vi "Artificial Horizon.vi"(7 "Fixed Camera Position":bool=TRUE, 8 "error in \n(no error)":errorcluster, 9 "Heading":dbl(slide) scale=-360.0..360.0, 10 "Roll":dbl(slide) scale=-180.0..180.0, 11 "Pitch":dbl(slide) scale=-90.0..90.0) -> (0 "error out":errorcluster, 3 "reference out":refnum<vi>(3d-picture))   [LabVIEW 2011]
doc: "Artificial Horizon.VI\n\nRecieves Pitch Roll and Head, and using a 3D picture control Builds up an artifical horizon similar to that found in aircraft for example."
uses:
  <vilib>/Utility/miscctls.llb/LV3DPointTypeDef.ctl
  <vilib>/picture/3D Picture Control/NI_3D Picture Control.lvlib
panel:
  in  "Stop Button":bool
  # "Disabled"
  # "Enabled"
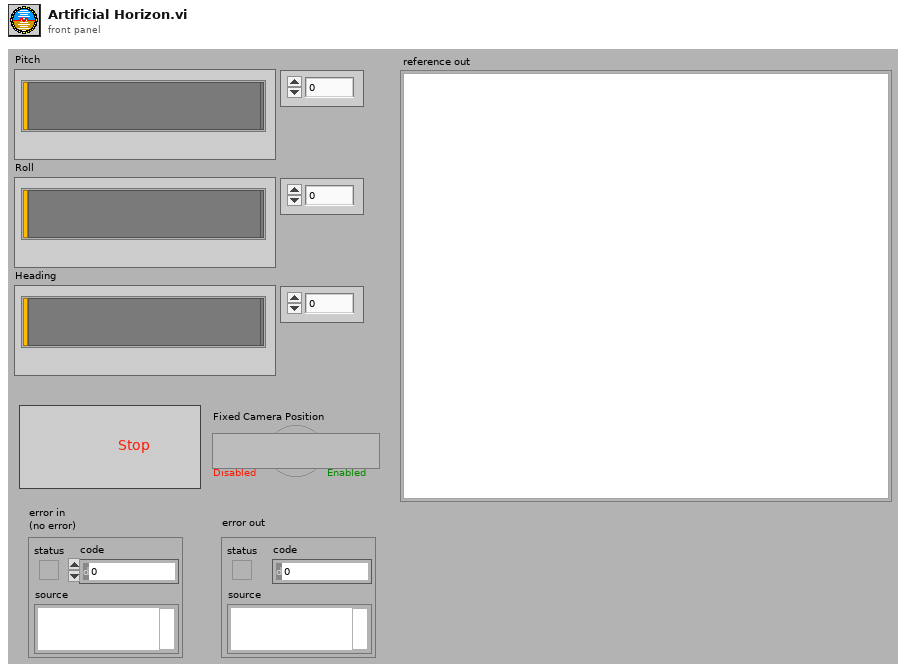
[diagram p1: front panel]
types:
  T1 = enum16{"None", "Spherical", "Flying", "Oriented"}
  T2 = typedef "LV3DPointTypeDef.ctl" = cluster{"X":sgl, "Y":sgl, "Z":sgl}
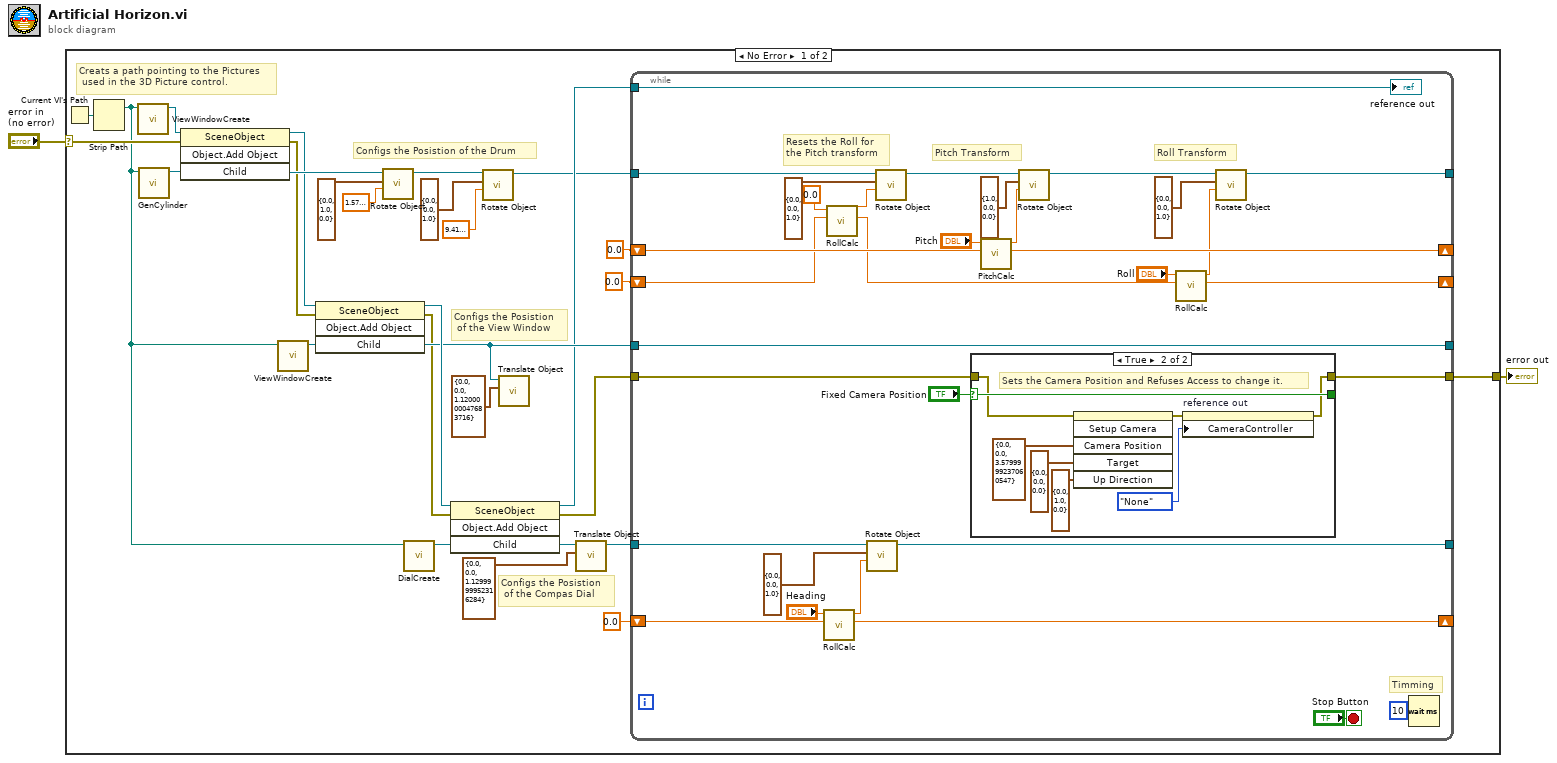
[diagram p0: block diagram]
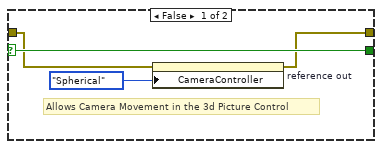
[diagram p2: hidden frame]
diagram:
  n1 = case shown="No Error" "error in \n(no error)" {
    selector: "error in \n(no error)" -> [w11 w76]
    tunnel: [w10 w76] -> w1
    frame No Error {
      # "Configs the Posistion\n of the Compas Dial"
      # "Configs the Posistion\n of the View Window"
      # "Configs the Posistion of the Drum"
      # "Creats a path pointing to the Pictures\n used in the 3D Picture control."
      n2 = Current VI's Path() -> (path=w6:path)
      n3 = Strip Path(path=w6) -> (stripped path=w4:path)  [unwired: 1 out]
      n4 = call "ViewWindowCreate.vi"("Solid Horizon Path.PNG"=w4) -> ("SceneObject out"=w5:refnum<vi>)  [unwired: 10 in]
      n5 = call "GenCylinder.vi"("Solid Horizon Path.PNG"=w4) -> ("SceneObject out"=w29:refnum<vi>)  [unwired: 10 in]
      n6 = invoke class="SceneObject" method="Object.Add Object"(reference=w5, error in=w11, "Child"=w29) -> (reference out=w15:refnum<vi>, error out=w9:errorcluster, "Child"=w22:refnum<vi>)  [unwired: 1 in, 1 out]
      n7 = call "ViewWindowCreate.vi"("Solid Horizon Path.PNG"=w4) -> ("SceneObject out"=w3:refnum<vi>)  [unwired: 10 in]
      n8 = invoke class="SceneObject" method="Object.Add Object"(reference=w15, error in=w9, "Child"=w3) -> (reference out=w31:refnum<vi>, error out=w8:errorcluster, "Child"=w25:refnum<vi>)  [unwired: 1 in, 1 out]
      n9 = call <vilib>:"Rotate Object.vi"("Angle"=sgl 1.5799999 ("Angle 2"), "Axis"=cluster{"X":sgl, "Y":sgl, "Z":sgl} {"X"=0.0, "Y"=1.0, "Z"=0.0} ("Axis 2"), "Scene.Object In"=w22) -> ("Scene.Object Out"=w21:refnum<vi>)  [unwired: 7 in, 1 out]
      n10 = call "DialCreate.vi"("Solid Horizon Path.PNG"=w4) -> ("SceneObject out"=w30:refnum<vi>)  [unwired: 10 in]
      n11 = invoke class="SceneObject" method="Object.Add Object"(reference=w31, error in=w8, "Child"=w30) -> (reference out=w16:refnum<vi>, error out=w7:errorcluster, "Child"=w26:refnum<vi>)  [unwired: 1 in, 1 out]
      n12 = call <vilib>:"Rotate Object.vi"("Angle"=sgl 9.419999 ("Angle 3"), "Axis"=cluster{"X":sgl, "Y":sgl, "Z":sgl} {"X"=0.0, "Y"=0.0, "Z"=1.0} ("Axis 3"), "Scene.Object In"=w21) -> ("Scene.Object Out"=w12:refnum<vi>)  [unwired: 7 in, 1 out]
      n13 = call <vilib>:"Translate Object.vi"("Translation"=cluster{"X":sgl, "Y":sgl, "Z":sgl} {"X"=0.0, "Y"=0.0, "Z"=1.12} ("Translation 4"), "Scene.Object In"=w25) -> ()  [unwired: 8 in, 2 out]
      n14 = call <vilib>:"Translate Object.vi"("Translation"=cluster{"X":sgl, "Y":sgl, "Z":sgl} {"X"=0.0, "Y"=0.0, "Z"=1.13} ("Translation 5"), "Scene.Object In"=w26) -> ("Scene.Object Out"=w14:refnum<vi>)  [unwired: 8 in, 1 out]
      n15 = while {
        tunnel: w25 -> [w58]
        tunnel: w16 -> [w62]
        tunnel: w12 -> [w61]
        shift-right: [w54] -> _
        shift-left: 0.0 ("y") -> [w55]
        shift-right: [w56] -> _
        shift-left: 0.0 ("y") -> [w52]
        tunnel: [w58] -> _
        tunnel: [w57] -> _
        tunnel: w14 -> [w50]
        shift-right: [w49] -> _
        shift-left: 0.0 ("y") -> [w51]
        tunnel: [w48] -> _
        tunnel: w7 -> [w34]
        tunnel: [w33] -> w10
        stop <- "Stop Button" stop-if-true
        # "Timming"
        # "Roll Transform"
        # "Resets the Roll for \nthe Pitch transform"
        # "Pitch Transform"
        n16 = call "RollCalc.vi"("Previous Roll Value"=w51, "Roll Input"="Heading") -> ("New Roll Value"=w49:dbl, "Adjustment to be Made"=w46:dbl)  [unwired: 8 in]
        n17 = call "RollCalc.vi"("Previous Roll Value"=w52, "Roll Input"=sgl 0.0 ("Angle")) -> ("New Roll Value"=w53:dbl, "Adjustment to be Made"=w40:dbl)  [unwired: 8 in]
        n18 = call <vilib>:"Rotate Object.vi"("Angle"=w46, "Axis"=cluster{"X":sgl, "Y":sgl, "Z":sgl} {"X"=0.0, "Y"=0.0, "Z"=1.0} ("Axis 2"), "Scene.Object In"=w50) -> ("Scene.Object Out"=w48:refnum<vi>)  [unwired: 7 in, 1 out]
        n19 = call <vilib>:"Rotate Object.vi"("Angle"=w40, "Axis"=cluster{"X":sgl, "Y":sgl, "Z":sgl} {"X"=0.0, "Y"=0.0, "Z"=1.0} ("Axis 2"), "Scene.Object In"=w61) -> ("Scene.Object Out"=w41:refnum<vi>)  [unwired: 7 in, 1 out]
        n20 = case shown="True" "Fixed Camera Position" {
          selector: "Fixed Camera Position" -> [w67 w72]
          tunnel: [w64 w68] -> w33
          tunnel: w34 -> [w66 w70]
          tunnel: [w67 w72] -> _
          frame False {
            # "Allows Camera Movement in the 3d Picture Control"
            n21 = property on="reference out" class="SceneGraphDisp (strict)"(error in=w66, "CameraController"=T1."Spherical" ("Camera Controller:Type")) -> (error out=w64:errorcluster)  [unwired: 1 in, 1 out]
          }
          frame True {
            # "Sets the Camera Position and Refuses Access to change it."
            n22 = invoke on="reference out" class="SceneGraphDisp (strict)" method="Setup Camera"(error in=w70, "Camera Position"=T2 {"X"=0.0, "Y"=0.0, "Z"=3.58}, "Target"=T2 {"X"=0.0, "Y"=0.0, "Z"=0.0}, "Up Direction"=T2 {"X"=0.0, "Y"=1.0, "Z"=0.0}) -> (error out=w69:errorcluster)  [unwired: 2 in, 5 out]
            n23 = property on="reference out" class="SceneGraphDisp (strict)"(error in=w69, "CameraController"=T1."None" ("Camera Controller:Type")) -> (error out=w68:errorcluster)  [unwired: 1 in, 1 out]
          }
        }
        n24 = call "PitchCalc.vi"("Previous Pitch Value"=w55, "Pitch Control"="Pitch") -> ("New Pitch Value"=w54:dbl, "Adjustment to be made"=w43:dbl)  [unwired: 8 in]
        n25 = call <vilib>:"Rotate Object.vi"("Angle"=w43, "Axis"=cluster{"X":sgl, "Y":sgl, "Z":sgl} {"X"=1.0, "Y"=0.0, "Z"=0.0} ("Axis 2"), "Scene.Object In"=w41) -> ("Scene.Object Out"=w59:refnum<vi>)  [unwired: 7 in, 1 out]
        n26 = call "RollCalc.vi"("Previous Roll Value"=w53, "Roll Input"="Roll") -> ("New Roll Value"=w56:dbl, "Adjustment to be Made"=w35:dbl)  [unwired: 8 in]
        n27 = call <vilib>:"Rotate Object.vi"("Angle"=w35, "Axis"=cluster{"X":sgl, "Y":sgl, "Z":sgl} {"X"=0.0, "Y"=0.0, "Z"=1.0} ("Axis 2"), "Scene.Object In"=w59) -> ("Scene.Object Out"=w57:refnum<vi>)  [unwired: 7 in, 1 out]
        n28 = Wait (ms)(milliseconds to wait=u32 10) -> ()  [unwired: 1 out]
        "reference out" <- w62
      }
    }
    frame Error {
      # "OOOOOOOOOOOOOOOOOOOOOOOOOOO NNNNNNNNNNNNNNNNnnnnnnnnnnnnnnnnooooooooooooooooooooooooooooooooo\n\nAn Error..........................................................."
    }
  }
  "error out" <- w1
